vi "wait on semaphores.vi"(8 "error in (no error)":errorcluster, 11 "semaphores in":T1[](array[typedef])) -> (0 "error out":errorcluster, 3 "semaphores out":T1[](array[typedef]))   [LabVIEW 2013, in "Shared Memory runtime.lvclass"]
uses:
  Shared Memory runtime.lvclass
  <vilib>/NI/Pthreads for LabVIEW on Linux RT/Classes/Semaphore/Controls/reference.ctl
  <vilib>/NI/Pthreads for LabVIEW on Linux RT/Classes/Semaphore/Semaphore.lvclass
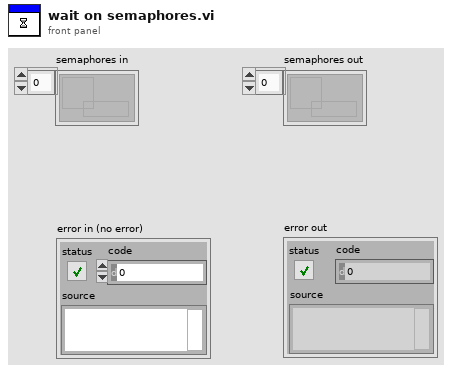
[diagram p1: front panel]
types:
  T1 = typedef "POSIX Threads.lvlib/Semaphore.lvclass/reference.ctl" = refnum<data-value>
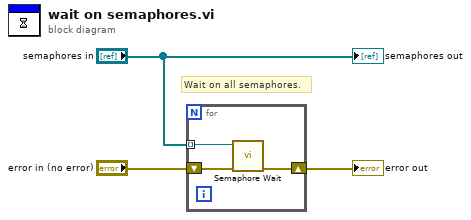
[diagram p0: block diagram]
diagram:
  # "Wait on all semaphores."
  n1 = for {
    shift-right: [w5] -> w2
    shift-left: "error in (no error)" -> [w6]
    tunnel: "semaphores in" -> [w4] mode=indexing
    n2 = call <vilib>:"Semaphore Wait.vi"("error in (no error)"=w6, "Semaphore in"=w4) -> ("error out"=w5:errorcluster)  [unwired: 8 in, 1 out]
  }
  "error out" <- w2
  "semaphores out" <- "semaphores in"
